vi "Run Client Stream.vi"(8 "error in":errorcluster, 10 "pin map context":T1, 11 "measurement configuration":T3) -> (0 "error out":errorcluster, 3 "measurement results":T2)   [LabVIEW 2021, in "Measurement Client Template.lvlib"]
doc: "<B>Run Client.vi</B> is a wrapper to demonstrate the working of Measurement Plug-In Client. It performs the following functions:\n- Create a client for the measurement service\n- Run the measurement logic and display the results\n- Close the client connection."
uses:
  controls/Measurement Configuration.ctl
  controls/Measurement Results.ctl
  <vilib>/gRPC/Generated APIs/ni/measurementlink/measurement/v2/Measurement Service Client V2/RPC Messages/ni_measurementlink_PinMapContext.ctl
  Measurement Client Template.lvlib
  <vilib>/gRPC/Generated APIs/ni/measurementlink/measurement/v2/Measurement Service Client V2/Measurement Service Client V2.lvlib
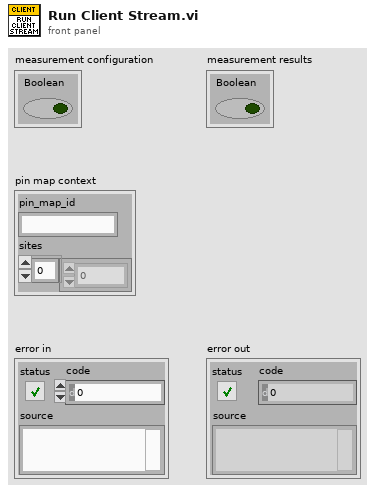
[diagram p1: front panel]
types:
  T1 = typedef "Measurement Service Client V2.lvlib/ni_measurementlink_PinMapContext.ctl" = cluster{"pin_map_id":string, "sites":i32[]}
  T2 = typedef "Measurement Client Template.lvlib/Measurement Results.ctl" = cluster{"Boolean":bool}
  T3 = typedef "Measurement Client Template.lvlib/Measurement Configuration.ctl" = cluster{"Boolean":bool}
  T4 = typedef "grpc-lvsupport-release.lvlib/grpcId.ctl" = u64
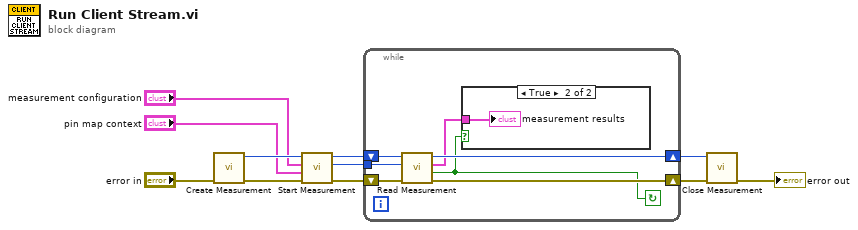
[diagram p0: block diagram]
diagram:
  n1 = call "Create Measurement.vi"("error in"="error in") -> ("error out"=w11:errorcluster, "gRPCid out"=w8:T4)  [unwired: 9 in]
  n2 = call "Start Measurement.vi"("error in"=w11, "pin map context"="pin map context", "measurement configuration"="measurement configuration", "gRPCid in"=w8) -> ("error out"=w9:errorcluster, "call id"=w4:T4, "gRPCid out"=w5:T4)  [unwired: 5 in]
  n3 = while {
    tunnel: w4 -> [w15]
    shift-right: [w17] -> w2
    shift-left: w9 -> [w18]
    shift-right: [w14] -> w3
    shift-left: w5 -> [w16]
    stop <- w12 continue-if-true
    n4 = call "Read Measurement.vi"("error in"=w18, "call id"=w15, "gRPCid in"=w16) -> ("error out"=w17:errorcluster, "measure success?"=w12:bool, "measurement results"=w13:T2, "gRPCid out"=w14:T4)  [unwired: 5 in]
    n5 = case shown="True" w12 {
      tunnel: w13 -> [_ w19]
      frame False {
      }
      frame True {
        "measurement results" <- w19
      }
    }
  }
  n6 = call "Close Measurement.vi"("error in"=w2, "gRPCid in"=w3) -> ("error out"=→"error out":errorcluster)  [unwired: 9 in]
